vi "Relay_PanelSim_Global.vi"(0 "menu":T4=enum."set init_rev", 5 "RelayChannel":T3, 7 "Value Set":bool, 11 "error in (no error)":errorcluster, 12 "String Value":string) -> (10 "Relay new":T1={"type"="Relay", "device"="", "name"="", "data"={"<init_fwd"=FALSE, "<init_rev"=FALSE, "<fwd"=FALSE, "<rev"=FALSE}}, 15 "error out":errorcluster)   [LabVIEW 2019]
doc: "This is used to set and get the last motor output values. This is needed for simulation, since we cannot read these values from the hardware.\n\nThis software is licensed. Open the labview\\readme\\WPI Robotics Library Open Source License.txt file for more information."
uses:
  Relay data proto.ctl
  Relay proto.ctl
  <vilib>/Rock Robotics/SystemInterfaces/DIO/FPGA_DIORelayChannel.ctl
  Relay Update Ops.ctl
panel:
  out "All Values":T1[](array[typedef])
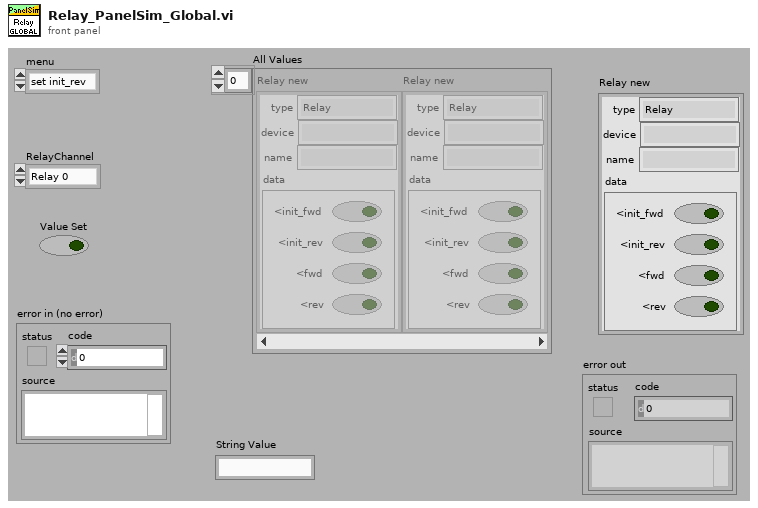
[diagram p1: front panel]
types:
  T1 = typedef "Relay proto.ctl" = cluster{"type":string, "device":string, "name":string, "data":T2}
  T2 = typedef "Relay data proto.ctl" = cluster{"<init_fwd":bool, "<init_rev":bool, "<fwd":bool, "<rev":bool}
  T3 = typedef "FPGA_DIORelayChannel.ctl" = enum8{"Relay 0", "Relay 1", "Relay 2", "Relay 3", "Invalid"}
  T4 = typedef "Relay Update Ops.ctl" = enum16{"set init_fwd", "set init_rev", "set fwd", "set rev", "get", "delete", "JSON update", "set name", "transmit initial", "reset"}
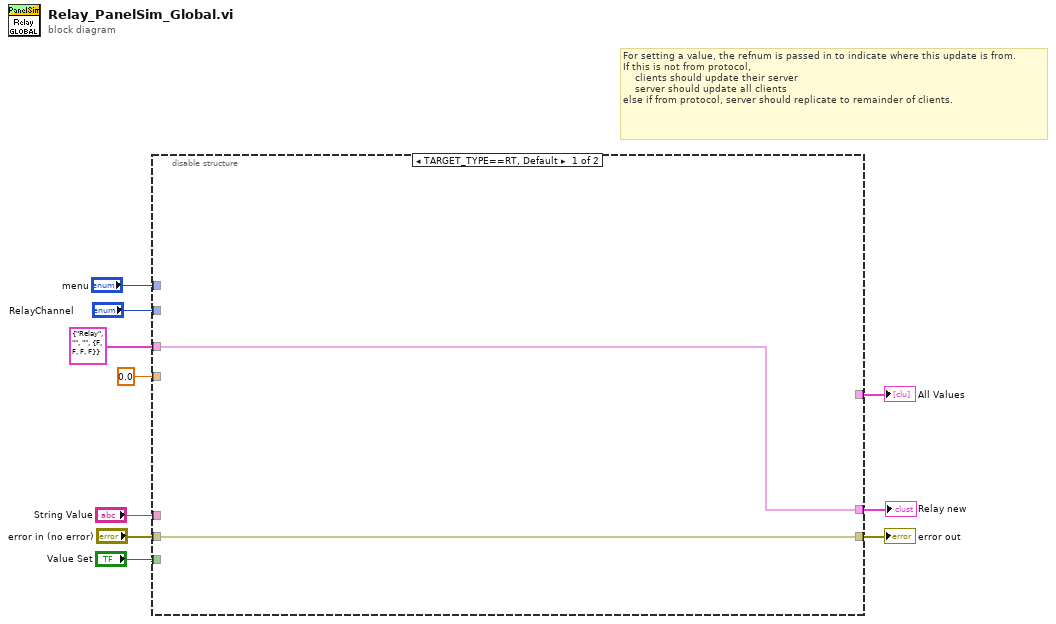
[diagram p0: block diagram]
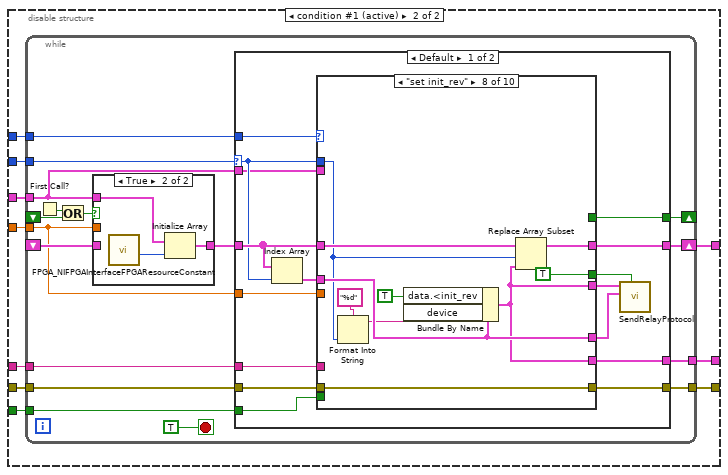
[diagram p2: hidden frame]
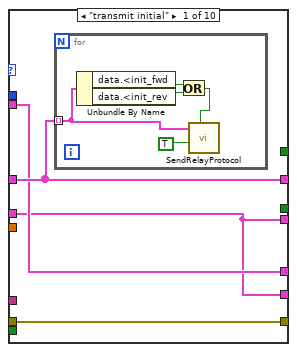
[diagram p3: hidden frame]
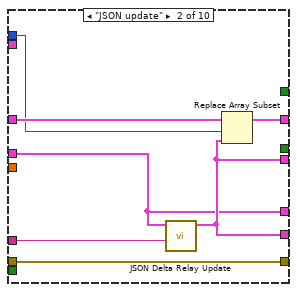
[diagram p4: hidden frame]
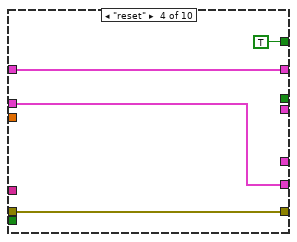
[diagram p6: hidden frame]
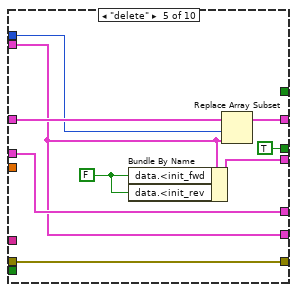
[diagram p7: hidden frame]
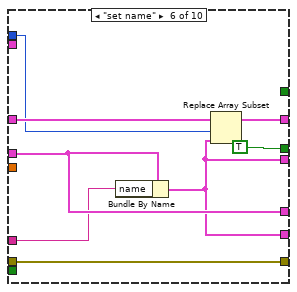
[diagram p8: hidden frame]
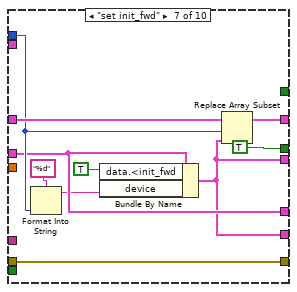
[diagram p9: hidden frame]
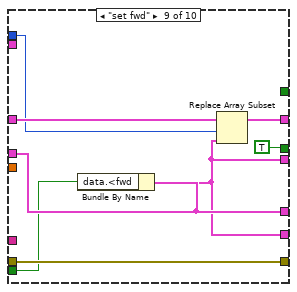
[diagram p10: hidden frame]
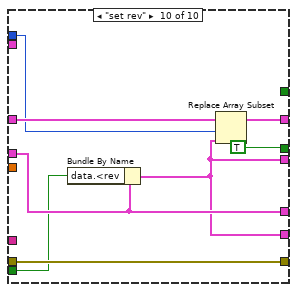
[diagram p11: hidden frame]
diagram:
  # "For setting a value, the refnum is passed in to indicate where this update is from.\nIf this is not from protocol,\n    clients should update their server\n    server should update all clients\nelse if from protocol, server should replicate to remainder of clients."
  n1 = disable-structure shown="TARGET_TYPE==RT, Default" {
    disable-tunnel: "menu" -> [_ w22]
    disable-tunnel: [w12 w21] -> w9
    disable-tunnel: "error in (no error)" -> [w12 w20]
    disable-tunnel: [_ w19] -> w7
    disable-tunnel: 0.0 ("Output") -> [_ w18]
    disable-tunnel: "RelayChannel" -> [_ w17]
    disable-tunnel: [w11 w16] -> w4
    disable-tunnel: T1 {"type"="Relay", "device"="", "name"="", "data"={"<init_fwd"=FALSE, "<init_rev"=FALSE, "<fwd"=FALSE, "<rev"=FALSE}} ("Relay new") -> [w11 w15]
    disable-tunnel: "String Value" -> [_ w14]
    disable-tunnel: "Value Set" -> [_ w13]
    frame condition #0 {
    }
    frame condition #1 (active) {
      n2 = while {
        tunnel: w20 -> [w36]
        shift-right: [w39] -> w19
        shift-left: _ -> [w32]
        tunnel: [w38] -> w16
        tunnel: w22 -> [w37]
        tunnel: [w35] -> w21
        tunnel: w17 -> [w30]
        tunnel: w18 -> [w31]
        tunnel: w15 -> [w29]
        tunnel: w14 -> [w28]
        tunnel: w13 -> [w27]
        shift-right: [w23] -> _
        shift-left: _ -> [w24]
        stop <- TRUE stop-if-true
        n3 = First Call?() -> (First Call?: T/F=w25:bool)
        n4 = Or(x=w25, y=w24) -> (x .or. y?=w26:bool)
        n5 = case shown="True" w26 {
          tunnel: [w135 w138] -> w33
          tunnel: w32 -> [w135 _]
          tunnel: w31 -> [_ _]
          tunnel: w29 -> [_ w136]
          frame False {
          }
          frame True {
            n6 = call <vilib>:"FPGA_NIFPGAInterfaceFPGAResourceConstant.vi"() -> ("NumberOfPWMs"=w137:u32)  [unwired: 11 out]
            n7 = Initialize Array(w136, w137) -> (w138:T1[])
          }
        }
        n8 = case shown="Default" w30 {
          selector: w30 -> [w48 _]
          tunnel: [w55 w134] -> w39
          tunnel: [w54 w132] -> w38
          tunnel: w37 -> [w53 _]
          tunnel: w36 -> [w52 w133]
          tunnel: [w51 w133] -> w35
          tunnel: w33 -> [w50 w134]
          tunnel: w31 -> [w49 _]
          tunnel: w29 -> [w46 w132]
          tunnel: w28 -> [w45 _]
          tunnel: w27 -> [w44 _]
          tunnel: [w40 _] -> w23
          frame Default {
            n9 = Index Array(array=w50, index=w48) -> (element=w47:T1)
            n10 = case shown="\"set init_rev\"" w53 {
              tunnel: [w58 w71 w74 w78 w86 w95 w105 w115 w123 w131] -> w55
              tunnel: w50 -> [w58 w69 w74 w78 w87 w93 w103 w113 w121 w129]
              tunnel: [w56 w67 w72 w76 w80 w89 w96 w110 w117 w125] -> w54
              tunnel: [w59 w70 w73 w77 w85 w94 w104 w114 w122 w130] -> w51
              tunnel: w52 -> [w59 w70 w73 w77 w85 w94 w104 w114 w122 w130]
              tunnel: w48 -> [_ w68 _ _ w82 w91 w100 w107 w119 w127]
              tunnel: w49 -> [_ _ _ _ _ _ _ _ _ _]
              tunnel: [w56 w67 _ _ w81 w89 w96 w110 w117 w125] -> w42
              tunnel: [w57 w66 _ _ w83 w90 w99 w111 w118 w126] -> w41
              tunnel: [_ _ _ _ TRUE TRUE TRUE TRUE TRUE TRUE] -> w43
              tunnel: w47 -> [w56 w66 w72 w76 w83 w90 w99 w111 w118 w126]
              tunnel: w46 -> [w57 _ _ _ w80 _ _ _ _ _]
              tunnel: w45 -> [_ w65 _ _ _ w88 _ _ _ _]
              tunnel: w44 -> [_ _ _ _ _ _ _ _ w116 w124]
              tunnel: [_ _ _ TRUE _ _ _ _ _ _] -> w40
              frame "transmit initial" {
                n11 = for {
                  tunnel: w58 -> [w64] mode=indexing
                  n12 = Unbundle By Name(w64) -> ("data.<init_fwd"=w62:bool, "data.<init_rev"=w61:bool)
                  n13 = Or(x=w62, y=w61) -> (x .or. y?=w60:bool)
                  n14 = call "SendRelayProtocol.vi"("Send"=w60, "Initialize"=TRUE, "Relay new"=w64) -> ()  [unwired: 9 in]
                }
              }
              frame "JSON update" {
                n15 = call "JSON Delta Relay Update.vi"("Delta JSON"=w65, "input"=w66) -> ("output"=w67:T1)  [unwired: 8 in, 1 out]
                n16 = Replace Array Subset(array=w69, new element=w67, index=w68) -> (w71:T1[])
              }
              frame "get" {
              }
              frame "reset" {
              }
              frame "delete" {
                w79 = FALSE ("data.<init_fwd")
                n17 = Bundle By Name(cluster=w80, "data.<init_fwd"=w79, "data.<init_rev"=w79) -> (w81:T1)
                n18 = Replace Array Subset(array=w87, new element=w80, index=w82) -> (w86:T1[])
              }
              frame "set name" {
                n19 = Bundle By Name(cluster=w90, "name"=w88) -> (w89:T1)
                n20 = Replace Array Subset(array=w93, new element=w89, index=w91) -> (w95:T1[])
              }
              frame "set init_fwd" {
                n21 = Format Into String(format string="%d", w100) -> (resulting string=w97:string)  [unwired: 2 in, 1 out]
                n22 = Bundle By Name(cluster=w99, "data.<init_fwd"=TRUE, "device"=w97) -> (w96:T1)
                n23 = Replace Array Subset(array=w103, new element=w96, index=w100) -> (w105:T1[])
              }
              frame "set init_rev" {
                n24 = Format Into String(format string="%d", w107) -> (resulting string=w106:string)  [unwired: 2 in, 1 out]
                n25 = Bundle By Name(cluster=w111, "data.<init_rev"=TRUE, "device"=w106) -> (w110:T1)
                n26 = Replace Array Subset(array=w113, new element=w110, index=w107) -> (w115:T1[])
              }
              frame "set fwd" {
                n27 = Bundle By Name(cluster=w118, "data.<fwd"=w116) -> (w117:T1)
                n28 = Replace Array Subset(array=w121, new element=w117, index=w119) -> (w123:T1[])
              }
              frame "set rev" {
                n29 = Bundle By Name(cluster=w126, "data.<rev"=w124) -> (w125:T1)
                n30 = Replace Array Subset(array=w129, new element=w125, index=w127) -> (w131:T1[])
              }
            }
            n31 = call "SendRelayProtocol.vi"("Send"=w43, "Relay prev"=w41, "Relay new"=w42) -> ()  [unwired: 9 in]
          }
          frame "Invalid" {
            # "Do nothing if \nchannel is Invalid."
          }
        }
      }
    }
  }
  "error out" <- w9
  "All Values" <- w7
  "Relay new" <- w4
